vi "Timing.Is Active Cycle.vi"(10 "iteration":u64=1, 11 "Timing in":refnum<class "Timing.lvclass">) -> (2 "active?":bool, 3 "Timing out":refnum<class "Timing.lvclass">)   [LabVIEW 2017, in "DSF.Engine.lvlib" / "Timing.lvclass"]
uses:
  Timing.lvclass
  Timing.lvclass/Timing.ctl
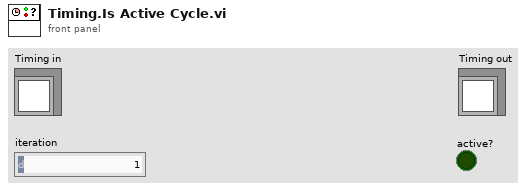
[diagram p1: front panel]
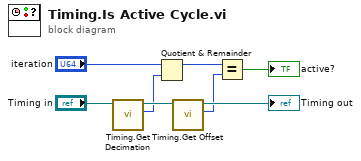
[diagram p0: block diagram]
diagram:
  n1 = call "Timing.Get Decimation.vi"("Timing in"="Timing in") -> ("Decimation"=w3:u64, "Timing out"=w7:refnum<class "Timing.lvclass">)  [unwired: 9 in]
  n2 = Quotient & Remainder(x="iteration", y=w3) -> (x-y*floor(x/y)=w6:u64)  [unwired: 1 out]
  n3 = call "Timing.Get Offset.vi"("Timing in"=w7) -> ("Offset"=w4:u64, "Timing out"=→"Timing out":refnum<class "Timing.lvclass">)  [unwired: 9 in]
  n4 = Equal?(x=w6, y=w4) -> (x = y?=→"active?":bool)
